vi "TestNoSubpanels.TestLauncher.vi"() -> ()   [LabVIEW 2020, in "TestNoSubpanels.lvclass"]
doc: "JKI State Machine Objects (SMO) 1.0.0.5\nJKI - JKI\nCopyright (c) 2016, JKI"
uses:
  TestNoSubpanels.lvclass
  C:/Program Files (x86)/National Instruments/LabVIEW 2020/vi.lib/JKI/JKI SMO/SMO/SMO.lvclass
  C:/Program Files (x86)/National Instruments/LabVIEW 2020/vi.lib/JKI/JKI SMO/SMO.UI/SMO.UI.lvclass
  <vilib>/JKI/JKI SMO/SMO/Typedefs/SMOState --Enum.ctl
  <vilib>/JKI/JKI SMO/SMO/SMO.lvclass
  <vilib>/JKI/JKI SMO/SMO.UI/SMO.UI.lvclass
  C:/Users/Albro/Documents/GitHub/MAUI-Engine/lvsrc/SMO.UI.MAUI.lvclass
  C:/Users/Albro/Documents/GitHub/MAUI-Engine/tests/relationship -- inheritance/TestInheritance/TestNoSubpanels.lvclass
panel:
  out "error out":errorcluster
  in  "Stop":bool
  # "TestNoSubpanels"
  # "For instructions on how to use the JKI State Machine Objects, examples and video tutorials, visit:\nhttp://jki.net/state-machine-objects/\n\nJKI State Machine Objects™\nhttp://jki.net/state-machine-objects/\nCopyright (C) 2005-2015, JKI <info@jki.net>\nALL RIGHTS RESERVED"
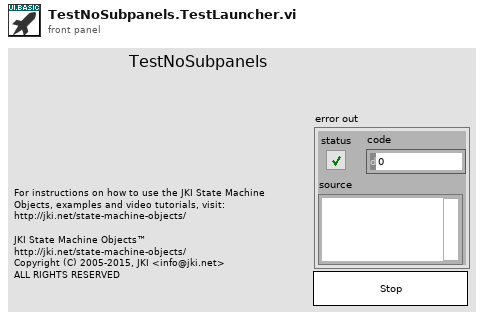
[diagram p1: front panel]
types:
  T1 = typedef "SMO.lvclass/Public Events.ctl" = cluster{"Error":refnum<user-event>, "State":refnum<user-event>, "Reserve State":refnum<user-event>}
  T2 = typedef "SMO.UI.lvclass/PublicEvents--Cluster.ctl" = cluster{"UI Hidden":refnum<user-event>, "UI State":refnum<user-event>}
  T3 = typedef "SMO.lvclass/SMOState --Enum.ctl" = enum16{"unknown", "Created", "Started", "Stopped"}
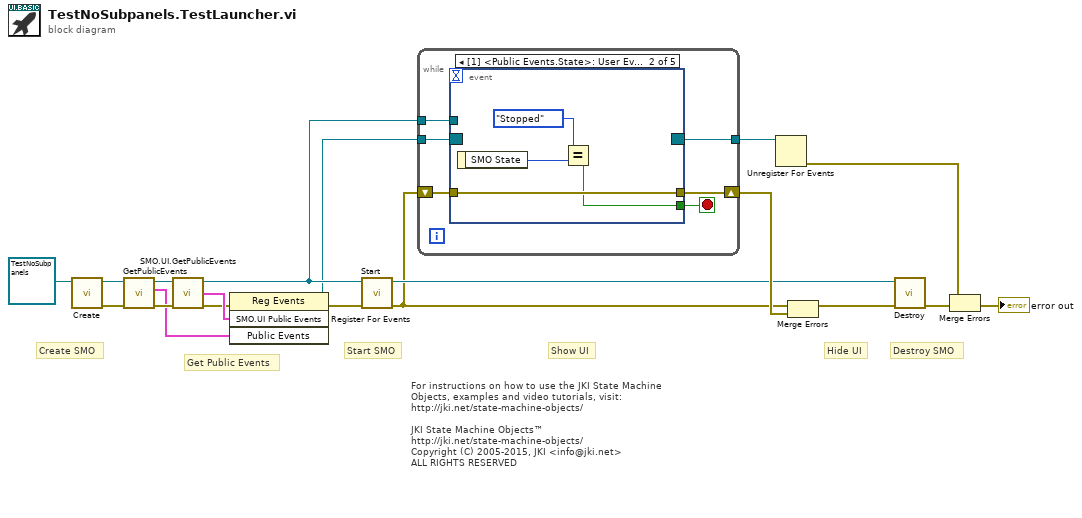
[diagram p0: block diagram]
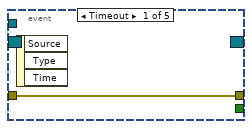
[diagram p2: hidden frame]
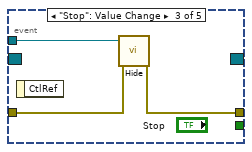
[diagram p3: hidden frame]
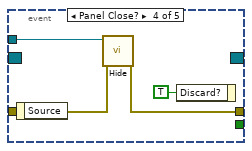
[diagram p4: hidden frame]
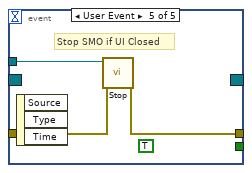
[diagram p5: hidden frame]
diagram:
  # "Hide UI"
  # "Show UI"
  # "For instructions on how to use the JKI State Machine Objects, examples and video tutorials, visit:\nhttp://jki.net/state-machine-objects/\n\nJKI State Machine Objects™\nhttp://jki.net/state-machine-objects/\nCopyright (C) 2005-2015, JKI <info@jki.net>\nALL RIGHTS RESERVED"
  # "Get Public Events"
  # "Start SMO"
  # "Destroy SMO"
  # "Create SMO"
  n1 = call <vilib>:"Create.vi"("SMO"=refnum<class "TestNoSubpanels.lvclass"> refnum ("SMO.Template.lvclass")) -> ("error out"=w7:errorcluster, "SMO out"=w6:refnum<class "TestNoSubpanels.lvclass">)  [unwired: 8 in, 1 out]
  n2 = call <vilib>:"GetPublicEvents.vi"("error in (no error)"=w7, "SMO"=w6) -> ("error out"=w4:errorcluster, "Public Events"=w3:T1, "SMO out"=w5:refnum<class "TestNoSubpanels.lvclass">)  [unwired: 7 in]
  n3 = call <vilib>:"SMO.UI.GetPublicEvents.vi"("error in (no error)"=w4, "SMO.UI"=w5) -> ("error out"=w10:errorcluster, "SMO.UI Public Events"=w11:T2, "SMO.UI out"=w12:refnum<class "TestNoSubpanels.lvclass">)  [unwired: 7 in]
  n4 = register-events(error in=w10, w11, w3) -> (reference out=w8:refnum<event-registration>, error out=w9:errorcluster)  [unwired: 1 in]
  n5 = call <vilib>:"Start.vi"("error in (no error)"=w9, "SMO"=w12) -> ("error out"=w1:errorcluster, "SMO out"=w2:refnum<class "TestNoSubpanels.lvclass">)  [unwired: 8 in]
  n6 = while {
    shift-right: [w24] -> w18
    shift-left: w1 -> [w23]
    tunnel: w8 -> [w22]
    tunnel: [w21] -> w19
    tunnel: w12 -> [w20]
    stop <- w25 stop-if-true
    n7 = event shown="[1] <Public Events.State>: User Event" {
      selector: w22 -> [_ _ _ _ _]
      dyn-events: [_ _ _ _ _] -> w21
      timeout: _ -> [_ _ _ _ _]
      tunnel: [_ w27 _ _ _] -> w25
      tunnel: w20 -> [_ _ w33 w36 w40]
      tunnel: [w26 w30 w31 w34 w39] -> w24
      tunnel: w23 -> [w26 w30 w32 w35 w38]
      event Timeout {
        n8 = event-data() -> ()  [unwired: 1 in, 3 out]
      }
      event User Event {
        n9 = event-data() -> ("SMO State"=w29:T3)  [unwired: 1 in]
        n10 = Equal?(x=SMOState_--Enum."Stopped", y=w29) -> (x = y?=w27:bool)
      }
      event "Stop": Value Change {
        n11 = event-data() -> ()  [unwired: 1 in, 1 out]
        n12 = call <vilib>:"Hide.vi"("error in (no error)"=w32, "SMO.UI"=w33) -> ("error out"=w31:errorcluster)  [unwired: 8 in, 1 out]
      }
      event Panel Close? {
        n13 = event-data() -> ()  [unwired: 1 in, 1 out]
        n14 = call <vilib>:"Hide.vi"("error in (no error)"=w35, "SMO.UI"=w36) -> ("error out"=w34:errorcluster)  [unwired: 8 in, 1 out]
        n15 = event-data("Discard?"=TRUE ("OK")) -> ()  [unwired: 1 in, 1 out]
      }
      event User Event {
        (unwired) TRUE ("OK")
        # "Stop SMO if UI Closed"
        n16 = event-data() -> ()  [unwired: 1 in, 3 out]
        n17 = call <vilib>:"Stop.vi"("error in (no error)"=w38, "SMO"=w40) -> ("error out"=w39:errorcluster)  [unwired: 8 in, 1 out]
      }
    }
  }
  n18 = Unregister For Events(event registration refnum=w19) -> (error out=w17:errorcluster)  [unwired: 1 in]
  n19 = Merge Errors(w1, w18) -> (w13:errorcluster)
  n20 = call <vilib>:"Destroy.vi"("error in (no error)"=w13, "SMO"=w2) -> ("error out"=w15:errorcluster)  [unwired: 9 in]
  n21 = Merge Errors(w17, w15) -> (→"error out":errorcluster)
